vi "XY Graph Pair Selected Plots Event.vi"(8 "Error In":errorcluster, 9 "Transpose?":bool, 11 "XYGraph Ref":T1) -> (0 "Error Out":errorcluster, 1 "Message":string)   [LabVIEW 2021, in "XY Graph Add-Ons.lvlib"]
uses:
  XY Graph Add-Ons.lvlib
  XY Graph Refnum.ctl
  XY Plot Data.ctl
  XY Graph Add Single Plot with Name.vi
  Strings/Strings.lvlib
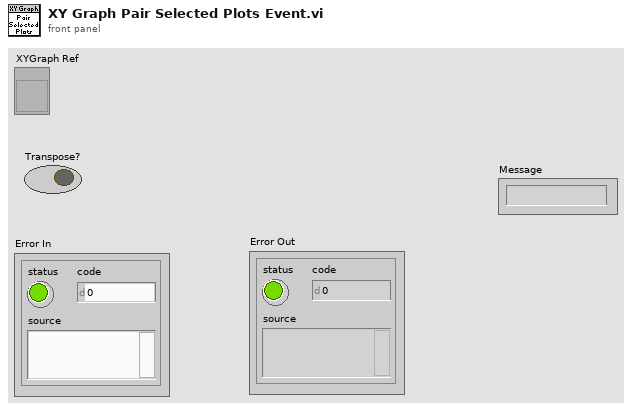
[diagram p1: front panel]
types:
  T1 = typedef "XY Graph Add-Ons.lvlib/XY Graph Refnum.ctl" = refnum<vi>
  T2 = typedef "XY Graph Add-Ons.lvlib/XY Plot Data.ctl" = cluster{"X Array":dbl[], "Y Array":dbl[]}
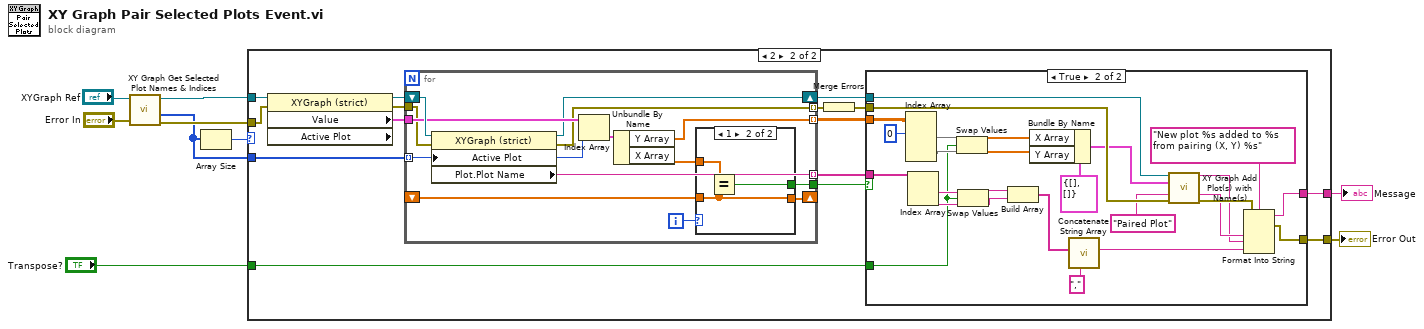
[diagram p0: block diagram]
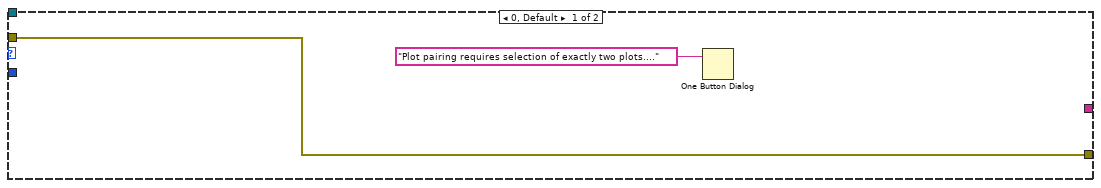
[diagram p2: hidden frame]
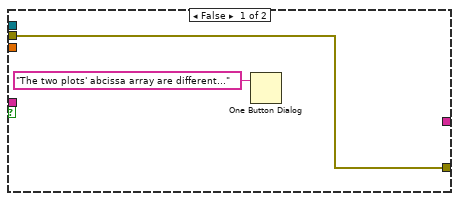
[diagram p3: hidden frame]
diagram:
  n1 = call "XY Graph Get Selected Plot Names & Indices.vi"("error in (no error)"="Error In", "XYGraph in"="XYGraph Ref") -> ("error out"=w6:errorcluster, "Selected Plots"=w5:i32[], "XYGraph out"=w7:T1)  [unwired: 5 in, 2 out]
  n2 = Array Size(array=w5) -> (size(s)=w4:i32)
  n3 = case shown="2" w4 {
    tunnel: w7 -> [_ w26]
    tunnel: w6 -> [w11 w25]
    tunnel: w5 -> [_ w20]
    tunnel: [_ w16] -> w3
    tunnel: [w11 w15] -> w2
    tunnel: "Transpose?" -> [_ w12]
    frame 0, Default {
      n4 = One Button Dialog(message="Plot pairing requires selection of exactly two plots....") -> ()  [unwired: 1 in, 1 out]
    }
    frame 2 {
      n5 = property class="XYGraph (strict)" props=["Value", "Active Plot"](reference=w26, error in=w25) -> (reference out=w24:T1, error out=w23:errorcluster, "Value"=w21:cluster{"X Array":dbl[], "Y Array":dbl[]}[])  [unwired: 1 out]
      n6 = for {
        tunnel: w20 -> [w65] mode=indexing
        tunnel: [w67] -> w18 mode=indexing
        tunnel: w21 -> [w66]
        shift-right: [w64] -> w17
        shift-left: w24 -> [w68]
        tunnel: w23 -> [w63]
        tunnel: [w62] -> w22 mode=indexing
        shift-right: [w59] -> _
        shift-left: _ -> [w58]
        tunnel: [w57] -> w14
        tunnel: [w55] -> w13 mode=indexing
        i -> [w61]
        n7 = property class="XYGraph (strict)"(reference=w68, error in=w63, "Active Plot"=w65) -> (reference out=w64:T1, error out=w62:errorcluster, "Plot.Plot Name"=w67:string)
        n8 = Index Array(array=w66, index=w65) -> (element=w56:cluster{"X Array":dbl[], "Y Array":dbl[]})
        n9 = Unbundle By Name(w56) -> ("Y Array"=w55:dbl[], "X Array"=w60:dbl[])
        n10 = case shown="1" w61 {
          tunnel: w60 -> [w69 w72]
          tunnel: [w69 w70] -> w59
          tunnel: w58 -> [_ w70]
          tunnel: [_ w71] -> w57
          frame 0, Default {
          }
          frame 1 {
            n11 = Equal?(x=w72, y=w70) -> (x = y?=w71:bool)
          }
        }
      }
      n12 = Merge Errors(w22) -> (w19:errorcluster)
      n13 = case shown="True" w14 {
        tunnel: w19 -> [w27 w53]
        tunnel: w18 -> [_ w35]
        tunnel: w17 -> [_ w51]
        tunnel: [_ w43] -> w16
        tunnel: [w27 w42] -> w15
        tunnel: w13 -> [_ w41]
        tunnel: w12 -> [_ w29]
        frame False {
          n14 = One Button Dialog(message="The two plots' abcissa array are different...") -> ()  [unwired: 1 in, 1 out]
        }
        frame True {
          n15 = Index Array(array=w41, index (row) #1=0 ("index (row)")) -> (element #1=w39:dbl[], element #2=w38:dbl[])  [unwired: 3 in]
          n16 = Index Array(array=w35) -> (element #1=w34:string, element #2=w33:string)  [unwired: 2 in]
          n17 = Swap Values(12:w39, 13:w29, 14:w38) -> (1:w37:dbl[], 3:w36:dbl[])
          n18 = Swap Values(12:w34, 13:w29, 14:w33) -> (1:w32:string, 3:w31:string)
          n19 = Build Array(w32, w31) -> (w30:string[])
          n20 = Bundle By Name(cluster=T2 {"X Array"=[], "Y Array"=[]} ("input cluster"), "X Array"=w37, "Y Array"=w36) -> (w50:T2)
          n21 = call "Concatenate String Array.vi"("Separator (TAB)"=",", "String Array"=w30) -> ("Formatted String"=w44:string)  [unwired: 9 in]
          n22 = call-poly "XY Graph Add Plot(s) with Name(s).vi"("XYGraph Ref in"=w51, "Plot"=w50, "Plot Name (\"Plot\")"="Paired Plot" ("Plot.Plot Name"), "error in (no error)"=w53) -> ("XY Graph Caption (or Label)"=w45:string, "Plot Name"=w46:string, "error out"=w48:errorcluster)  [unwired: 8 in, 1 out]
          n23 = Format Into String(format string="New plot %s added to %s from pairing (X, Y) %s", error in=w48, w46, w45, w44) -> (resulting string=w43:string, error out=w42:errorcluster)  [unwired: 1 in]
        }
      }
    }
  }
  "Error Out" <- w2
  "Message" <- w3
